vi "StopMotion.vi"(8 "error in":errorcluster, 11 "condition":i32) -> (0 "error out":errorcluster)   [LabVIEW 2013]
uses:
  NIST2/Arm Globals.vi
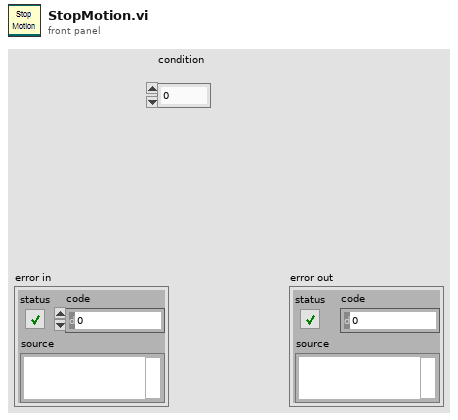
[diagram p1: front panel]
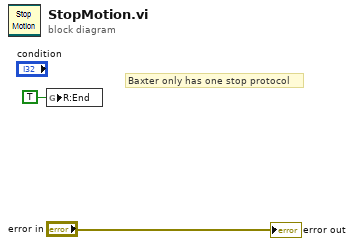
[diagram p0: block diagram]
diagram:
  # "Baxter only has one stop protocol"
  n1 = global write "Arm Globals.vi" "R:End"(TRUE ("R:End")) -> ()
  "error out" <- "error in"
